vi "Clear.vi"(8 "error in (no error)":errorcluster, 10 "Control":T1, 11 "Cluster":T2) -> (0 "error out":errorcluster)   [LabVIEW 2025, in "Test Unit.lvlib"]
uses:
  Test Unit.lvlib
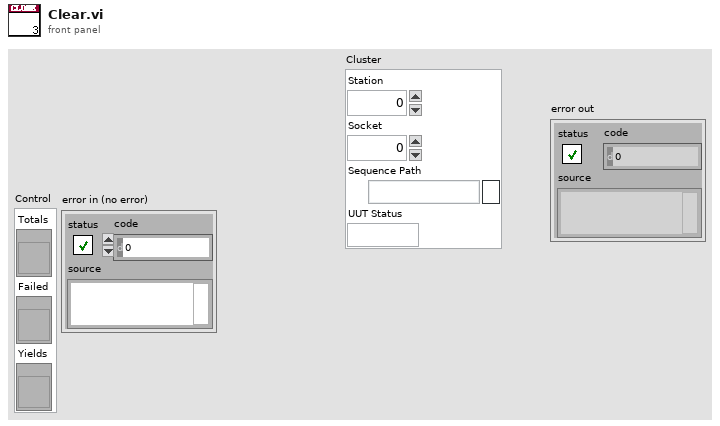
[diagram p1: front panel]
types:
  T1 = cluster{"Totals":refnum<vi>, "Failed":refnum<vi>, "Yields":refnum<vi>}
  T2 = cluster{"Station":i32, "Socket":i32, "Sequence Path":path, "UUT Status":string}
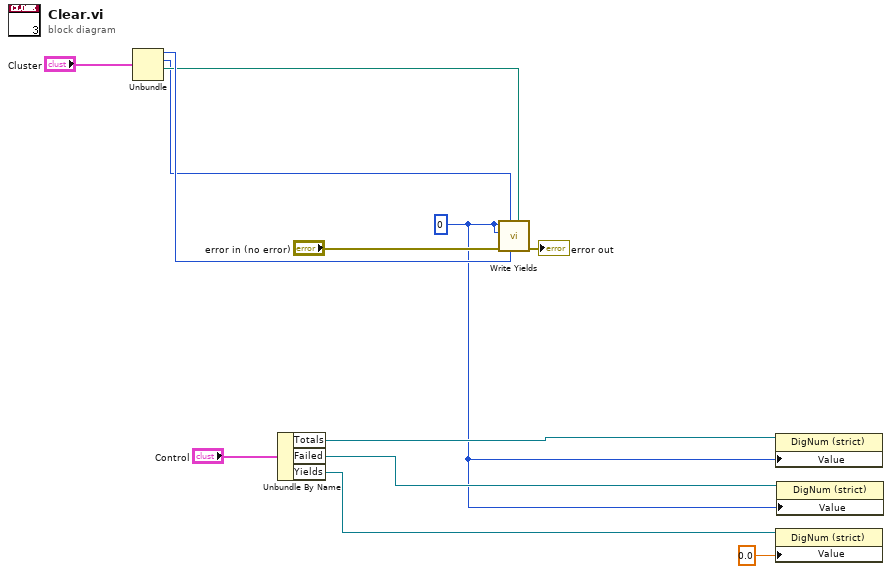
[diagram p0: block diagram]
diagram:
  w2 = 0 ("Totals")
  n1 = Unbundle("Cluster") -> ("Station"=w6:i32, "Socket"=w4:i32, "Sequence Path"=w5:path)  [unwired: 1 out]
  n2 = Unbundle By Name("Control") -> ("Totals"=w11:refnum<vi>, "Failed"=w10:refnum<vi>, "Yields"=w9:refnum<vi>)
  n3 = call "Write Yields.vi"("General.Sequence Path"=w5, "Station"=w6, "Socket"=w4, "error in (no error)"="error in (no error)", "Failed"=w2, "Totals"=w2) -> ("error out"=→"error out":errorcluster)  [unwired: 5 in]
  n4 = property class="DigNum (strict)"(reference=w11, "Value"=w2) -> ()  [unwired: 1 in, 2 out]
  n5 = property class="DigNum (strict)"(reference=w9, "Value"=0.0) -> ()  [unwired: 1 in, 2 out]
  n6 = property class="DigNum (strict)"(reference=w10, "Value"=w2) -> ()  [unwired: 1 in, 2 out]
